vi "scripting polymorphic.vi"() -> ()   [LabVIEW 2020]
panel:
  out "Array":path[](array[path])
  out "resulting string":string
  out "concatenated string":string
  out "InstanceInfo":T1(array[cluster])
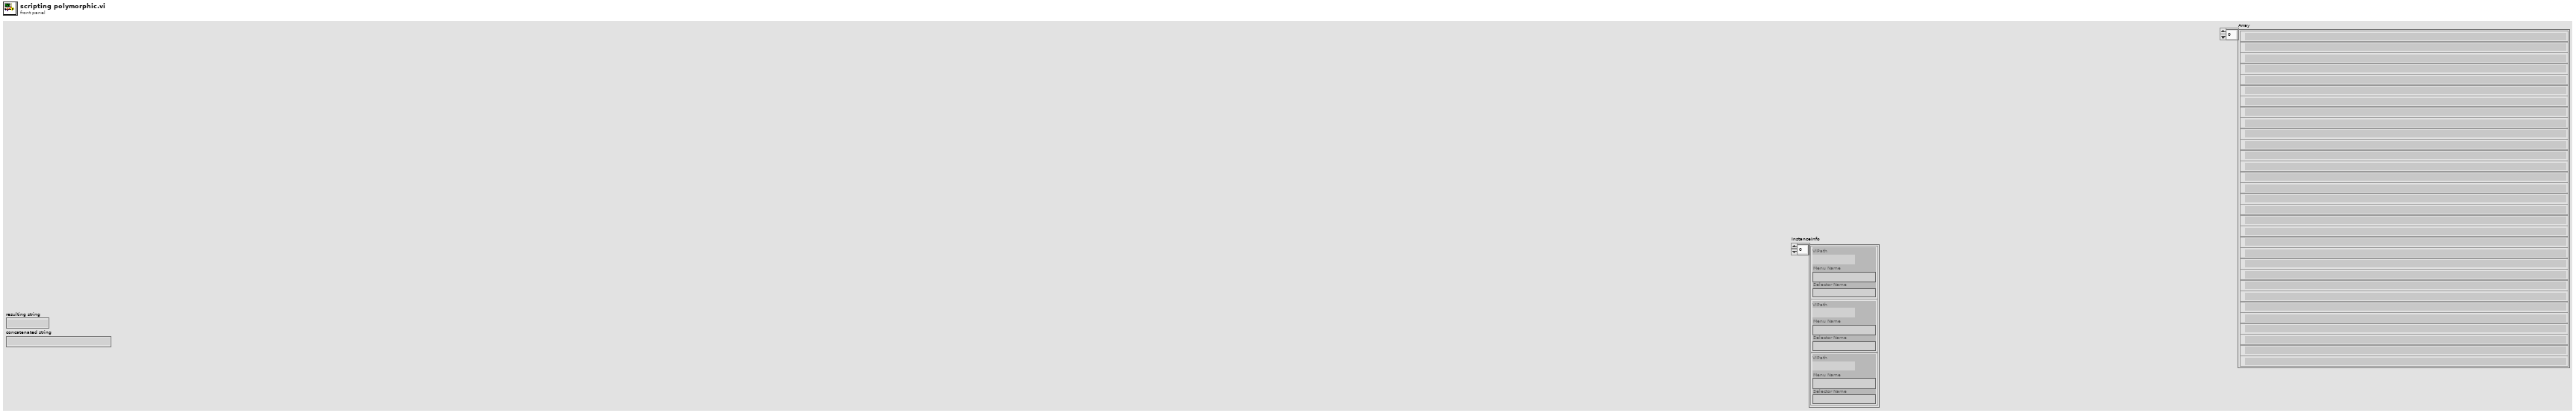
[diagram p1: front panel]
types:
  T1 = cluster{"VIPath":path, "Menu Name":string, "Selector Name":string}[]
  T2 = cluster{"VIPath":path, "Menu Name":string, "Selector Name":string}
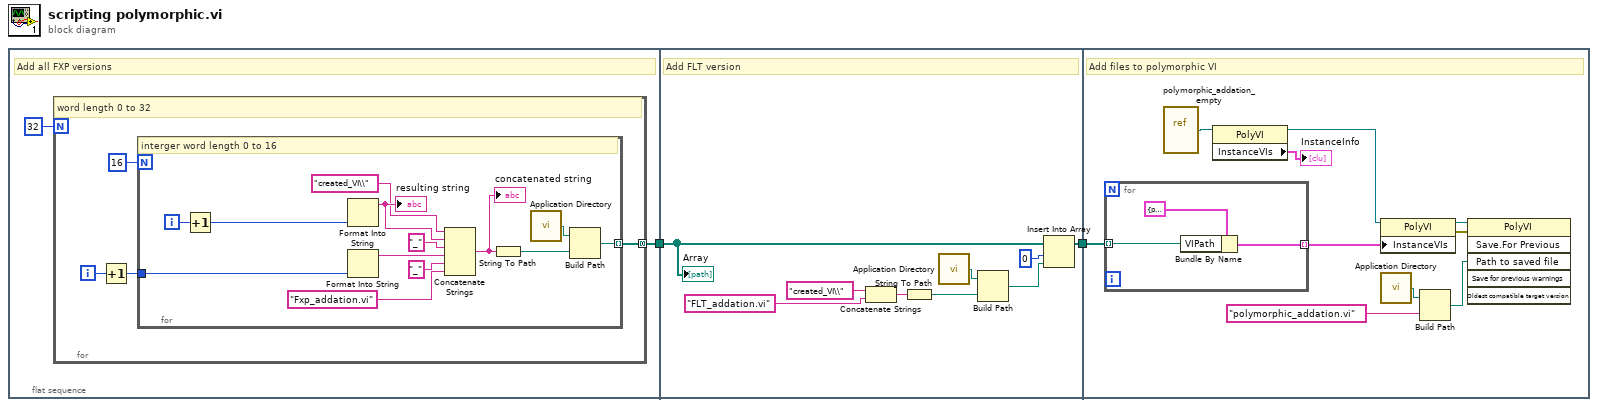
[diagram p0: block diagram]
diagram:
  n1 = flat-sequence {
    tunnel: [w3] -> w1
    tunnel: [w22] -> w2
    tunnel: w1 -> [w23]
    tunnel: w2 -> [w32]
    frame #0 {
      # "Add all FXP versions"
      n2 = for {
        N: 32 -> [_]
        tunnel: [w5] -> w3 mode=concatenating
        i -> [w8]
        # "word length 0 to 32"
        n3 = Increment(x=w8) -> (x+1=w6:i32)
        n4 = for {
          N: 16 -> [_]
          tunnel: w6 -> [w21]
          tunnel: [w9] -> w5 mode=indexing
          i -> [w19]
          # "interger word length 0 to 16"
          n5 = Increment(x=w19) -> (x+1=w20:i32)
          n6 = Format Into String(w20) -> (resulting string=w16:string)  [unwired: 3 in, 1 out]
          "resulting string" <- w16
          n7 = Format Into String(w21) -> (resulting string=w17:string)  [unwired: 3 in, 1 out]
          n8 = Concatenate Strings("created_VI\\" ("string"), w16, "_" ("string"), w17, "_" ("string"), "Fxp_addation.vi" ("string")) -> (w10:string)
          "concatenated string" <- w10
          n9 = String To Path(string=w10) -> (path=w18:path)
          n10 = call <vilib>:"Application Directory.vi"() -> ("Application Directory"=w15:path)
          n11 = Build Path(base path=w15, name or relative path=w18) -> (appended path=w9:path)
        }
      }
    }
    frame #1 {
      # "Add FLT version"
      n12 = Concatenate Strings("created_VI\\" ("string"), "FLT_addation.vi" ("string")) -> (w29:string)
      n13 = String To Path(string=w29) -> (path=w28:path)
      n14 = call <vilib>:"Application Directory.vi"() -> ("Application Directory"=w27:path)
      n15 = Build Path(base path=w27, name or relative path=w28) -> (appended path=w30:path)
      n16 = Insert Into Array(array=w23, index=0, new element=w30) -> (w22:path[])
      "Array" <- w23
    }
    frame #2 {
      # "Add files to polymorphic VI"
      n17 = for {
        tunnel: [w43] -> w40 mode=indexing
        tunnel: w32 -> [w42] mode=indexing
        n18 = Bundle By Name(cluster=T2 {"VIPath"=path "", "Menu Name"="", "Selector Name"=""}, "VIPath"=w42) -> (w43:T2)
      }
      n19 = vi-ref "polymorphic_addation_empty.vi"() -> (w31:refnum<vi>)
      n20 = property class="PolyVI"(reference=w31) -> (reference out=w38:refnum<vi>, "InstanceVIs"=→"InstanceInfo":T1)  [unwired: 1 in, 1 out]
      n21 = property class="PolyVI"(reference=w38, "InstanceVIs"=w40) -> (reference out=w34:refnum<vi>, error out=w33:errorcluster)  [unwired: 1 in]
      n22 = call <vilib>:"Application Directory.vi"() -> ("Application Directory"=w36:path)
      n23 = Build Path(base path=w36, name or relative path="polymorphic_addation.vi" ("string")) -> (appended path=w35:path)
      n24 = invoke class="PolyVI" method="Save.For Previous"(reference=w34, error in=w33, "Path to saved file"=w35) -> ()  [unwired: 3 in, 6 out]
    }
  }
